vi "Delete Empty Directories.vi"(8 "error in (no error)":errorcluster, 11 "Path":path) -> (0 "error out":errorcluster, 3 "folders removed":path[](array[path]))   [LabVIEW 2024]
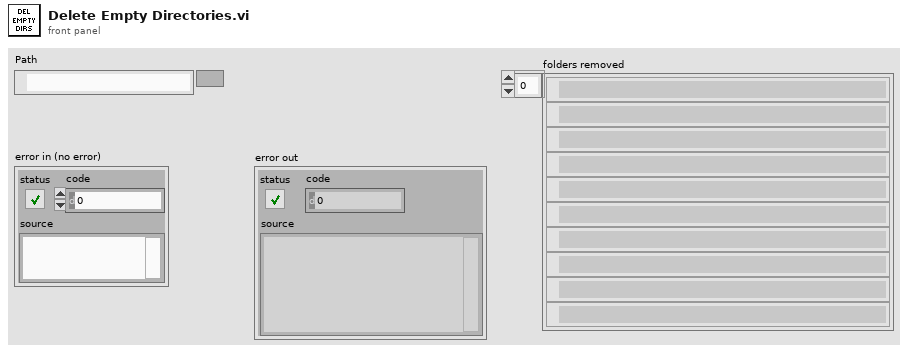
[diagram p1: front panel]
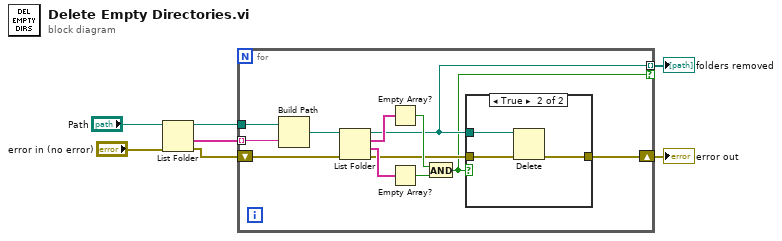
[diagram p0: block diagram]
diagram:
  n1 = List Folder(path="Path", error in="error in (no error)") -> (path out=w6:path, folder names=w5:string[], error out=w4:errorcluster)  [unwired: 2 in, 1 out]
  n2 = for {
    tunnel: w6 -> [w19]
    tunnel: w5 -> [w18] mode=indexing
    shift-right: [w10] -> w3
    shift-left: w4 -> [w16]
    tunnel: [w9] -> w2 mode=indexing if=w8
    n3 = Build Path(base path=w19, name or relative path=w18) -> (appended path=w17:path)
    n4 = List Folder(path=w17, error in=w16) -> (path out=w9:path, filenames=w15:string[], folder names=w14:string[], error out=w11:errorcluster)  [unwired: 2 in]
    n5 = Empty Array?(array=w15) -> (empty?=w12:bool)
    n6 = Empty Array?(array=w14) -> (empty?=w13:bool)
    n7 = And(x=w12, y=w13) -> (x .and. y?=w8:bool)
    n8 = case shown="True" w8 {
      tunnel: w11 -> [w20 w23]
      tunnel: w9 -> [_ w22]
      tunnel: [w20 w21] -> w10
      frame False {
      }
      frame True {
        n9 = Delete(path (use dialog)=w22, error in=w23) -> (error out=w21:errorcluster)  [unwired: 3 in, 2 out]
      }
    }
  }
  "error out" <- w3
  "folders removed" <- w2
